vi "BallSensors.vi"(3 "MinDistance(in.)":dbl, 5 "BallSensorDevRefIn":T1 {"Handle" format="%x"}) -> (0 "BallThere?":bool, 1 "Distance(in.)":dbl, 2 "OffsetFromCenter(in.)":dbl)   [LabVIEW 2019]
uses:
  <vilib>/Playing With Fusion Inc/Playing With Fusion Lib for FRC/PWF_ToF_LabVIEW/Public/TypeDefs/PwF_ToF_DevRef.ctl
  <vilib>/Playing With Fusion Inc/Playing With Fusion Lib for FRC/PWF_ToF_LabVIEW/PwF_ToF.lvlib
panel:
  in  "Threshold(in.)":dbl=5.0
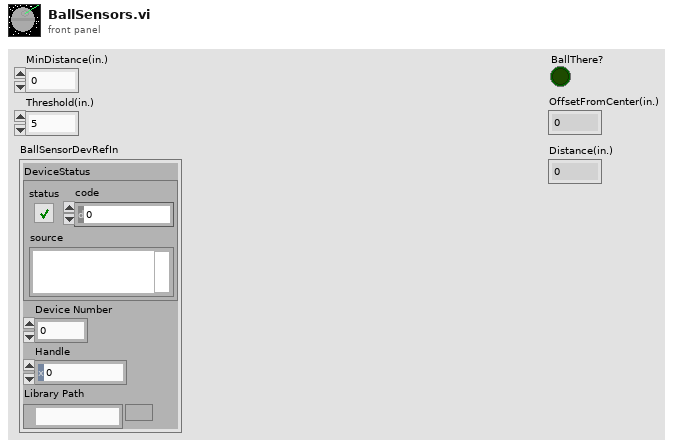
[diagram p1: front panel]
types:
  T1 = typedef "PlayingWithFusionLib.lvlib/PwF_ToF.lvlib/PwF_ToF_DevRef.ctl" = cluster{"DeviceStatus":errorcluster, "Device Number":u8, "Handle":u64, "Library Path":path}
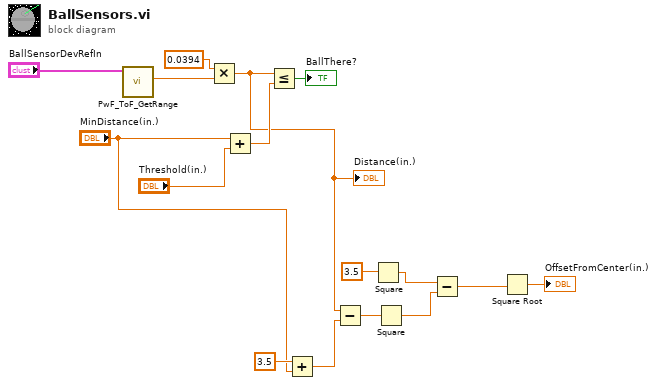
[diagram p0: block diagram]
diagram:
  n1 = call <vilib>:"PwF_ToF_GetRange.vi"("PwFToFDevRefIn"="BallSensorDevRefIn") -> ("range (mm)"=w16:dbl)  [unwired: 8 in, 2 out]
  n2 = Multiply(x=0.0394, y=w16) -> (x*y=w1:dbl)
  "Distance(in.)" <- w1
  n3 = Add(x="MinDistance(in.)", y="Threshold(in.)") -> (x+y=w13:dbl)
  n4 = Less Or Equal?(x=w1, y=w13) -> (x <= y?=→"BallThere?":bool)
  n5 = Add(x=3.5, y="MinDistance(in.)") -> (x+y=w10:dbl)
  n6 = Subtract(x=w1, y=w10) -> (x-y=w9:dbl)
  n7 = Square(x=3.5) -> (x^2=w7:dbl)
  n8 = Square(x=w9) -> (x^2=w6:dbl)
  n9 = Subtract(x=w7, y=w6) -> (x-y=w5:dbl)
  n10 = Square Root(x=w5) -> (sqrt(x)=→"OffsetFromCenter(in.)":dbl)
